vi "Run Action_Do.vi"(8 "error in (no error)":errorcluster, 10 "Project Builder in":refnum<class "Project Builder.lvclass">, 11 "PPL Class Test":refnum<class "PPL Class Test.lvclass">) -> (0 "error out":errorcluster, 1 "Success?":bool, 3 "Report":refnum<class "Report Data.lvclass">)   [LabVIEW 2019, in "ProjectBuilder.lvlib" / "PPL Class Test.lvclass"]
doc: "Run the action associated with the 'Project Action'-class.\n\nThis implementation load tests classes in PPL(s)."
uses:
  PPL Class Test.lvclass
  Data/Report Data/Report Data.lvclass
  Project Builder/Project Builder.lvclass
  PPL Class Test.lvclass/PPL Class Test.ctl
  PPL Class Test Data/PPL Class Test Data.lvclass/PPL Class Test Data.ctl
  PPL Class Test Data/PPL Class Test Data.lvclass
  C:/WS/prev/LV32.2019..ProjectBuilder/Class/Data/Report Data/Report Data.lvclass
  <vilib>/Utility/error.llb/Error Cluster From Error Code.vi
  <vilib>/ErrorRing/Error Ring.xnode
  ProjectBuilder.lvlib
  PPL/HDH.ClassLoader.lvlibp
  PPL Class Test Plugin/PPL Class Test Plugin.lvclass
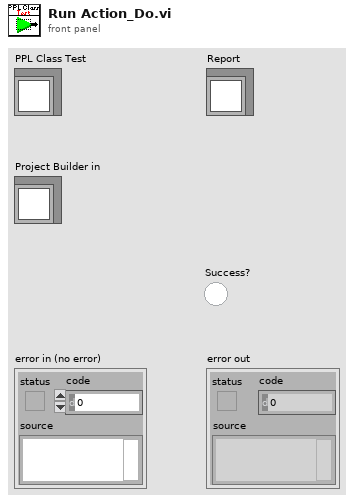
[diagram p1: front panel]
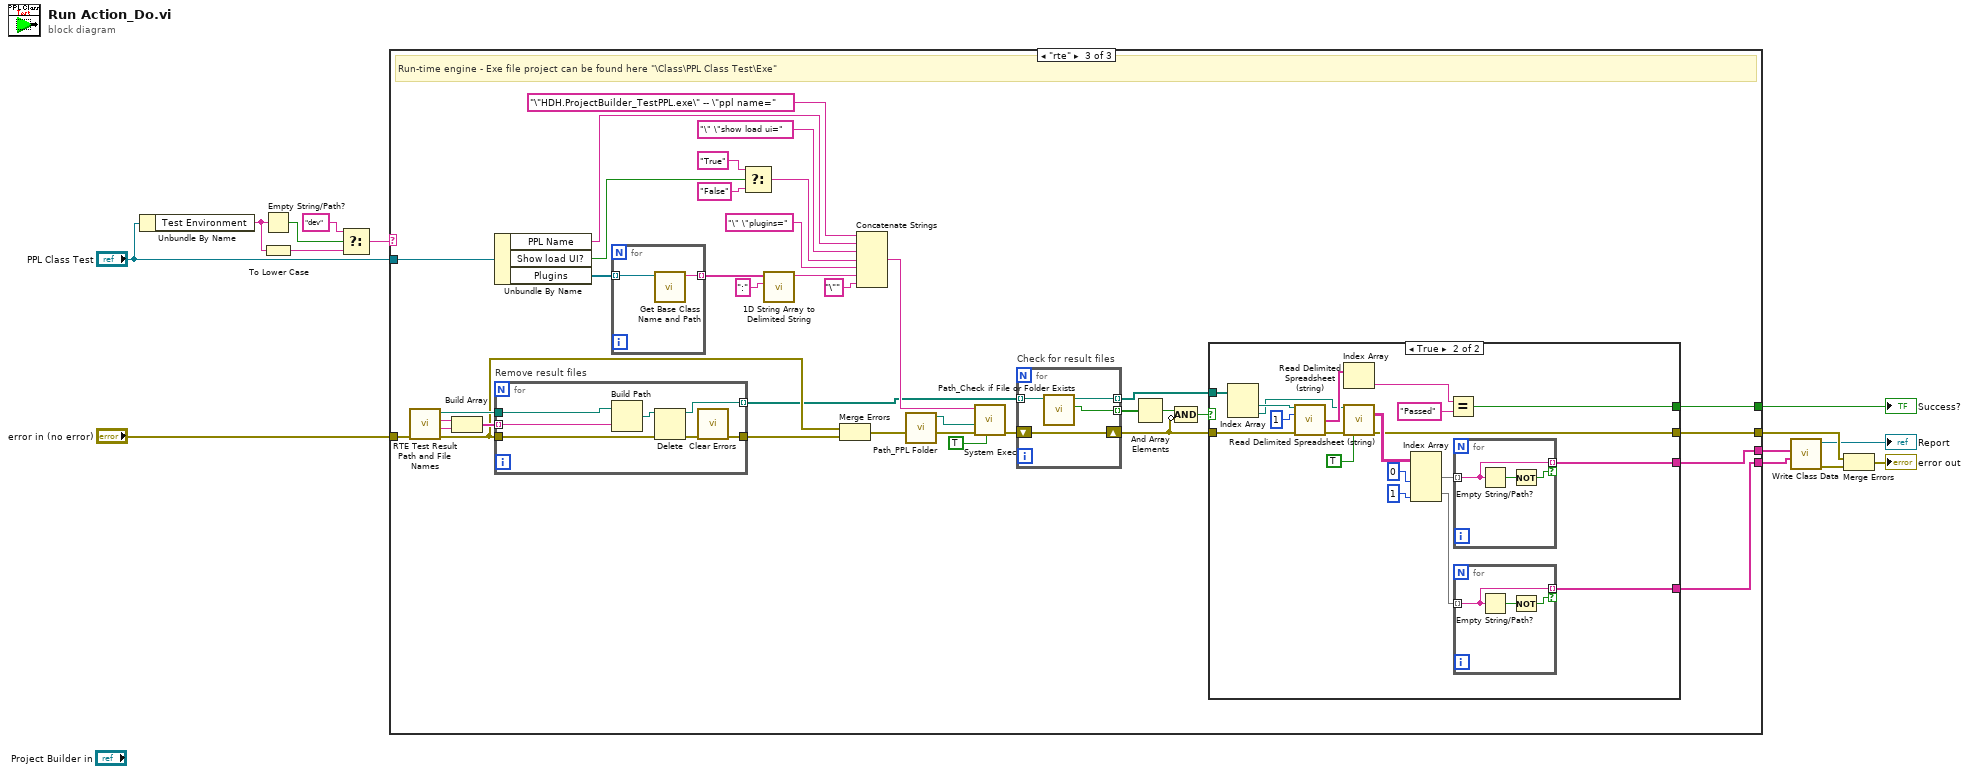
[diagram p0: block diagram]
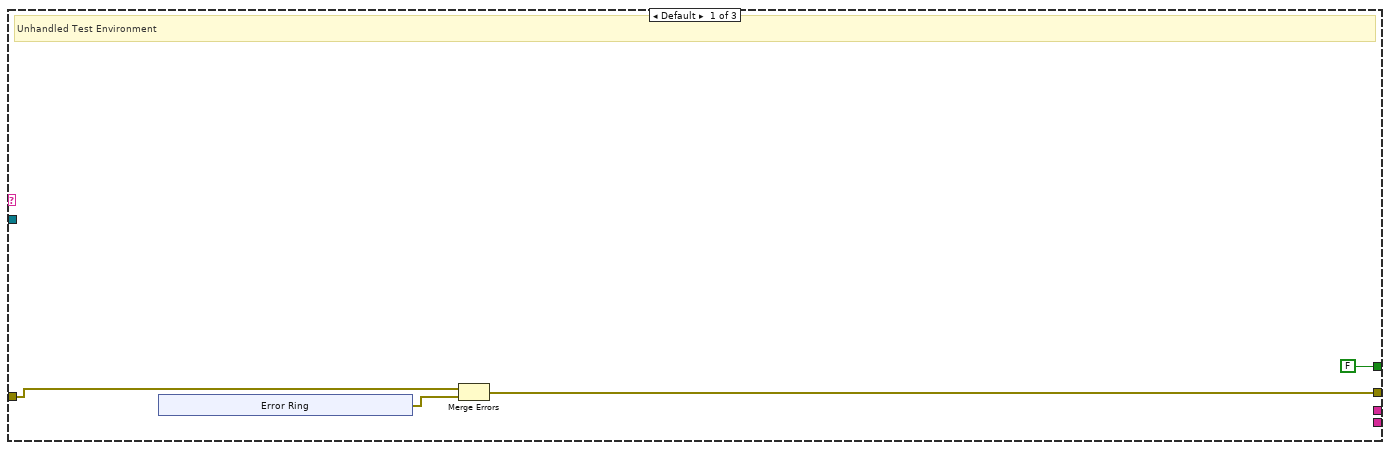
[diagram p2: hidden frame]
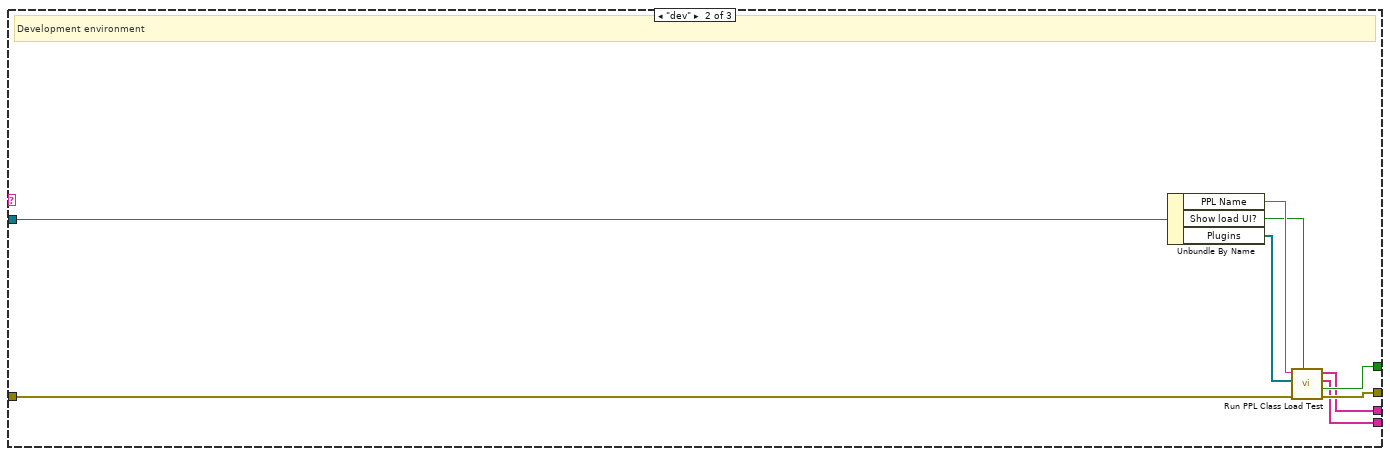
[diagram p3: hidden frame]
diagram:
  n1 = Unbundle By Name("PPL Class Test") -> ("Test Environment"=w13:string)
  n2 = Empty String/Path?(string/path=w13) -> (empty?=w14:bool)
  n3 = To Lower Case(string=w13) -> (all lower case string=w11:string)
  n4 = Select(t="dev", s=w14, f=w11) -> (s? t:f=w10:string)
  n5 = case shown="\"rte\"" w10 {
    tunnel: "error in (no error)" -> [w18 w29 w65]
    tunnel: [w16 w28 w35] -> w8
    tunnel: [FALSE w27 w36] -> w7
    tunnel: "PPL Class Test" -> [_ w31 w60]
    tunnel: [_ w26 w33] -> w3
    tunnel: [_ w25 w32] -> w2
    frame Default {
      # "Unhandled Test Environment"
      n6 = xnode "Error Ring"() -> ("error out"=w15:errorcluster)
      n7 = Merge Errors(w18, w15) -> (w16:errorcluster)
    }
    frame "dev" {
      # "Development environment"
      n8 = Unbundle By Name(w31) -> ("PPL Name"=w30:string, "Show load UI?"=w24:bool, "Plugins"=w23:refnum<class "PPL Class Test Plugin.lvclass">[])
      n9 = call "Run PPL Class Load Test.vi"("Show UI on Class load?(T)"=w24, "error in"=w29, "PPL Class Test Plugins"=w23, "PPL Name in PPL folder (entire PPL folder if empty)"=w30) -> ("error out"=w28:errorcluster, "Success?"=w27:bool, "Load Failure"=w25:string[], "Load Success"=w26:string[])  [unwired: 4 in]
    }
    frame "rte" {
      # "Run-time engine - Exe file project can be found here \"\\Class\\PPL Class Test\\Exe\""
      n10 = call "RTE Test Result Path and File Names.vi"("error in (no error)"=w65) -> ("error out"=w61:errorcluster, "PPL Test_Strings.txt"=w64:string, "PPL Test_Status.txt"=w67:string, "HDH\\ProjectBuilder\\temp path"=w66:path)  [unwired: 7 in]
      n11 = Build Array(w67, w64) -> (w63:string[])
      n12 = Unbundle By Name(w60) -> ("PPL Name"=w58:string, "Show load UI?"=w55:bool, "Plugins"=w56:refnum<class "PPL Class Test Plugin.lvclass">[])
      n13 = for "Remove result files" {
        tunnel: w66 -> [w107]
        tunnel: w63 -> [w106] mode=indexing
        tunnel: w61 -> [w104]
        tunnel: [w102] -> w62
        tunnel: [w101] -> w41 mode=indexing
        n14 = Build Path(base path=w107, name or relative path=w106) -> (appended path=w105:path)
        n15 = Delete(path (use dialog)=w105, error in=w104) -> (deleted path=w101:path, error out=w103:errorcluster)  [unwired: 3 in, 1 out]
        n16 = call <vilib>:"Clear Errors.vi"("error in (no error)"=w103) -> ("error out"=w102:errorcluster)  [unwired: 5 in, 1 out]
      }
      n17 = for {
        tunnel: w56 -> [w100] mode=indexing
        tunnel: [w99] -> w50 mode=indexing
        n18 = call "Get Base Class Name and Path.vi"("Class"=w100) -> ("Base Class Name"=w99:string)  [unwired: 8 in, 2 out]
      }
      n19 = Select(t="True", s=w55, f="False") -> (s? t:f=w52:string)
      n20 = call <vilib>:"1D String Array to Delimited String.vi"("delimiter"=":", "string array"=w50) -> ("delimited string"=w48:string)  [unwired: 9 in]
      n21 = Merge Errors(w61, w62) -> (w44:errorcluster)
      n22 = Concatenate Strings("\"HDH.ProjectBuilder_TestPPL.exe\" -- \"ppl name=" ("string"), w58, "\" \"show load ui=" ("string"), w52, "\" \"plugins=" ("string"), w48, "\"" ("string")) -> (w46:string)
      n23 = call "Path_PPL Folder.vi"() -> ("Data Folder Path"=w45:path)  [unwired: 10 in, 1 out]
      n24 = call <vilib>:"System Exec.vi"("run minimized? (F)"=TRUE, "error in (no error)"=w44, "working directory"=w45, "command line"=w46) -> ("error out"=w42:errorcluster)  [unwired: 4 in, 3 out]
      n25 = for "Check for result files" {
        tunnel: w41 -> [w71] mode=indexing
        shift-right: [w70] -> w34
        shift-left: w42 -> [w70]
        tunnel: [w69] -> w37 mode=indexing
        tunnel: [w68] -> w40 mode=indexing
        n26 = call "Path_Check if File or Folder Exists.vi"("File or Folder Path in"=w71) -> ("File or Folder Found?"=w68:bool, "File or Folder Path dub"=w69:path)  [unwired: 9 in]
      }
      n27 = And Array Elements(Boolean array=w40) -> (logical AND=w39:bool)
      n28 = Compound Arithmetic op=AND(w39, invert w34) -> (w38:bool)
      n29 = case shown="True" w38 {
        selector: w38 -> [w73 _]
        tunnel: w37 -> [_ w92]
        tunnel: [w73 w89] -> w36
        tunnel: [w72 w75] -> w35
        tunnel: w34 -> [w72 w85]
        tunnel: [_ w78] -> w33
        tunnel: [_ w76] -> w32
        frame False {
        }
        frame True {
          n30 = Index Array(array=w92) -> (element #1=w88:path, element #2=w83:path)  [unwired: 2 in]
          n31 = call <vilib>:"Read Delimited Spreadsheet (string).vi"("file path (dialog if empty)"=w88, "number of rows (all:-1)"=1, "error in (no error)"=w85) -> ("first row"=w86:string[], "error out"=w84:errorcluster)  [unwired: 7 in, 4 out]
          n32 = Index Array(array=w86) -> (element=w91:string)  [unwired: 1 in]
          n33 = call <vilib>:"Read Delimited Spreadsheet (string).vi"("file path (dialog if empty)"=w83, "error in (no error)"=w84, "transpose? (F)"=TRUE) -> ("all rows"=w82:string[][], "error out"=w75:errorcluster)  [unwired: 7 in, 4 out]
          n34 = Index Array(array=w82, index (col) #1=0 ("disabled index (col)"), index (col) #2=1 ("index (col)")) -> (element #1=w79:string[], element #2=w77:string[])  [unwired: 2 in]
          n35 = Equal?(x=w91, y="Passed") -> (x = y?=w89:bool)
          n36 = for {
            tunnel: w79 -> [w97] mode=indexing
            tunnel: [w97] -> w78 mode=indexing if=w96
            n37 = Empty String/Path?(string/path=w97) -> (empty?=w98:bool)
            n38 = Not(x=w98) -> (.not. x?=w96:bool)
          }
          n39 = for {
            tunnel: w77 -> [w94] mode=indexing
            tunnel: [w94] -> w76 mode=indexing if=w93
            n40 = Empty String/Path?(string/path=w94) -> (empty?=w95:bool)
            n41 = Not(x=w95) -> (.not. x?=w93:bool)
          }
        }
      }
    }
  }
  "Success?" <- w7
  n42 = call "Write Class Data.vi"("Load Failure"=w2, "Load Success"=w3) -> ("error out"=w4:errorcluster, "PPL Class Test Data out"=→"Report":refnum<class "PPL Class Test Data.lvclass">)  [unwired: 8 in]
  n43 = Merge Errors(w8, w4) -> (→"error out":errorcluster)
